vi "Read Data.vi"(8 "error in (no error)":errorcluster, 11 "Database in":refnum<class "Database.lvclass">) -> (0 "error out":errorcluster, 2 "DatabaseReadData":T1, 3 "Database out":refnum<class "Database.lvclass">)   [LabVIEW 2022 SP3, in "Database.lvclass"]
doc: "Developed by Kevin Thompson\nkevin@thompsonengineering.net\n\nCopyright 2018\nThompson Engineering, LLC"
uses:
  Database.lvclass
  DataTypes/Read Data--cluster.ctl
  Database.lvclass/Database.ctl
  Accessors/Set ReadData.vi
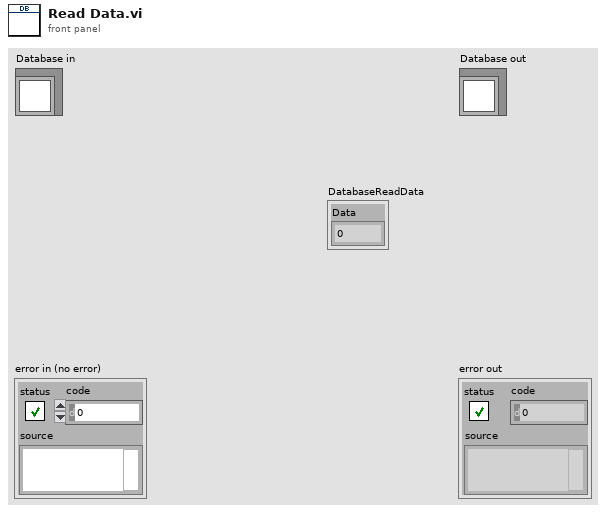
[diagram p1: front panel]
types:
  T1 = typedef "Database.lvclass/Read Data--cluster.ctl" = cluster{"Data":dbl}
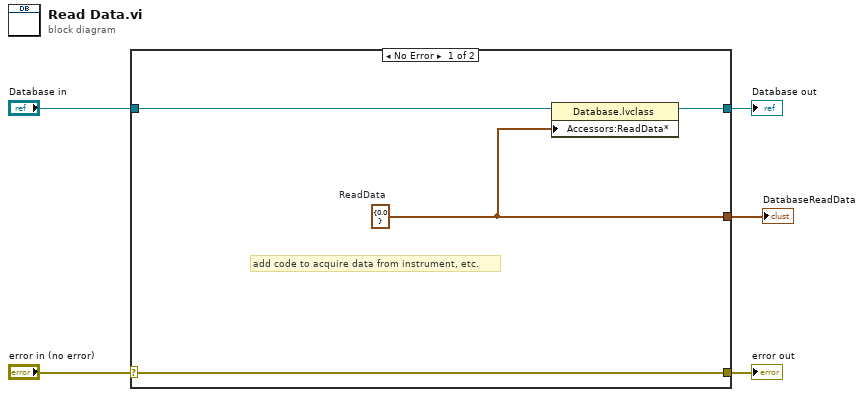
[diagram p0: block diagram]
diagram:
  n1 = case shown="No Error" "error in (no error)" {
    selector: "error in (no error)" -> [w9 w11]
    tunnel: [w9 w11] -> w4
    tunnel: [w7 w10] -> w2
    tunnel: "Database in" -> [w8 w10]
    tunnel: [w6 _] -> w1
    frame No Error {
      w6 = T1 {"Data"=0.0}  # ReadData
      # "add code to acquire data from instrument, etc."
      n2 = property class="Database.lvclass"(reference=w8, "Accessors:ReadData*"=w6) -> (reference out=w7:refnum<class "Database.lvclass">)  [unwired: 1 in, 1 out]
    }
    frame Error {
    }
  }
  "error out" <- w4
  "Database out" <- w2
  "DatabaseReadData" <- w1
